vi "User@CallVIWait__Parameter.vi"(1 "ParamterIn":string) -> (0 "ParamterOut":string)   [LabVIEW 2019]
uses:
  MainFrame/Global.vi
panel:
  in  "VI":string(combo)
  in  "Confirm":bool
  # "User@CallVIWait $VI"
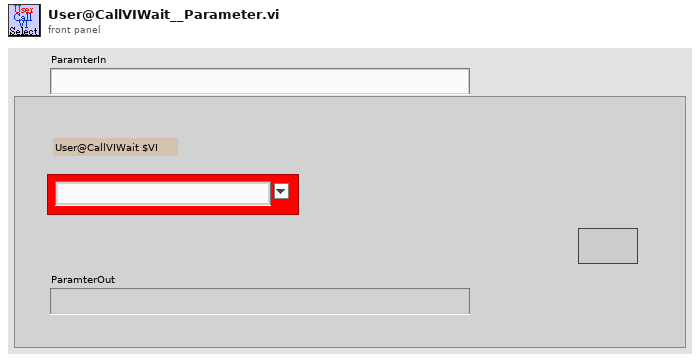
[diagram p1: front panel]
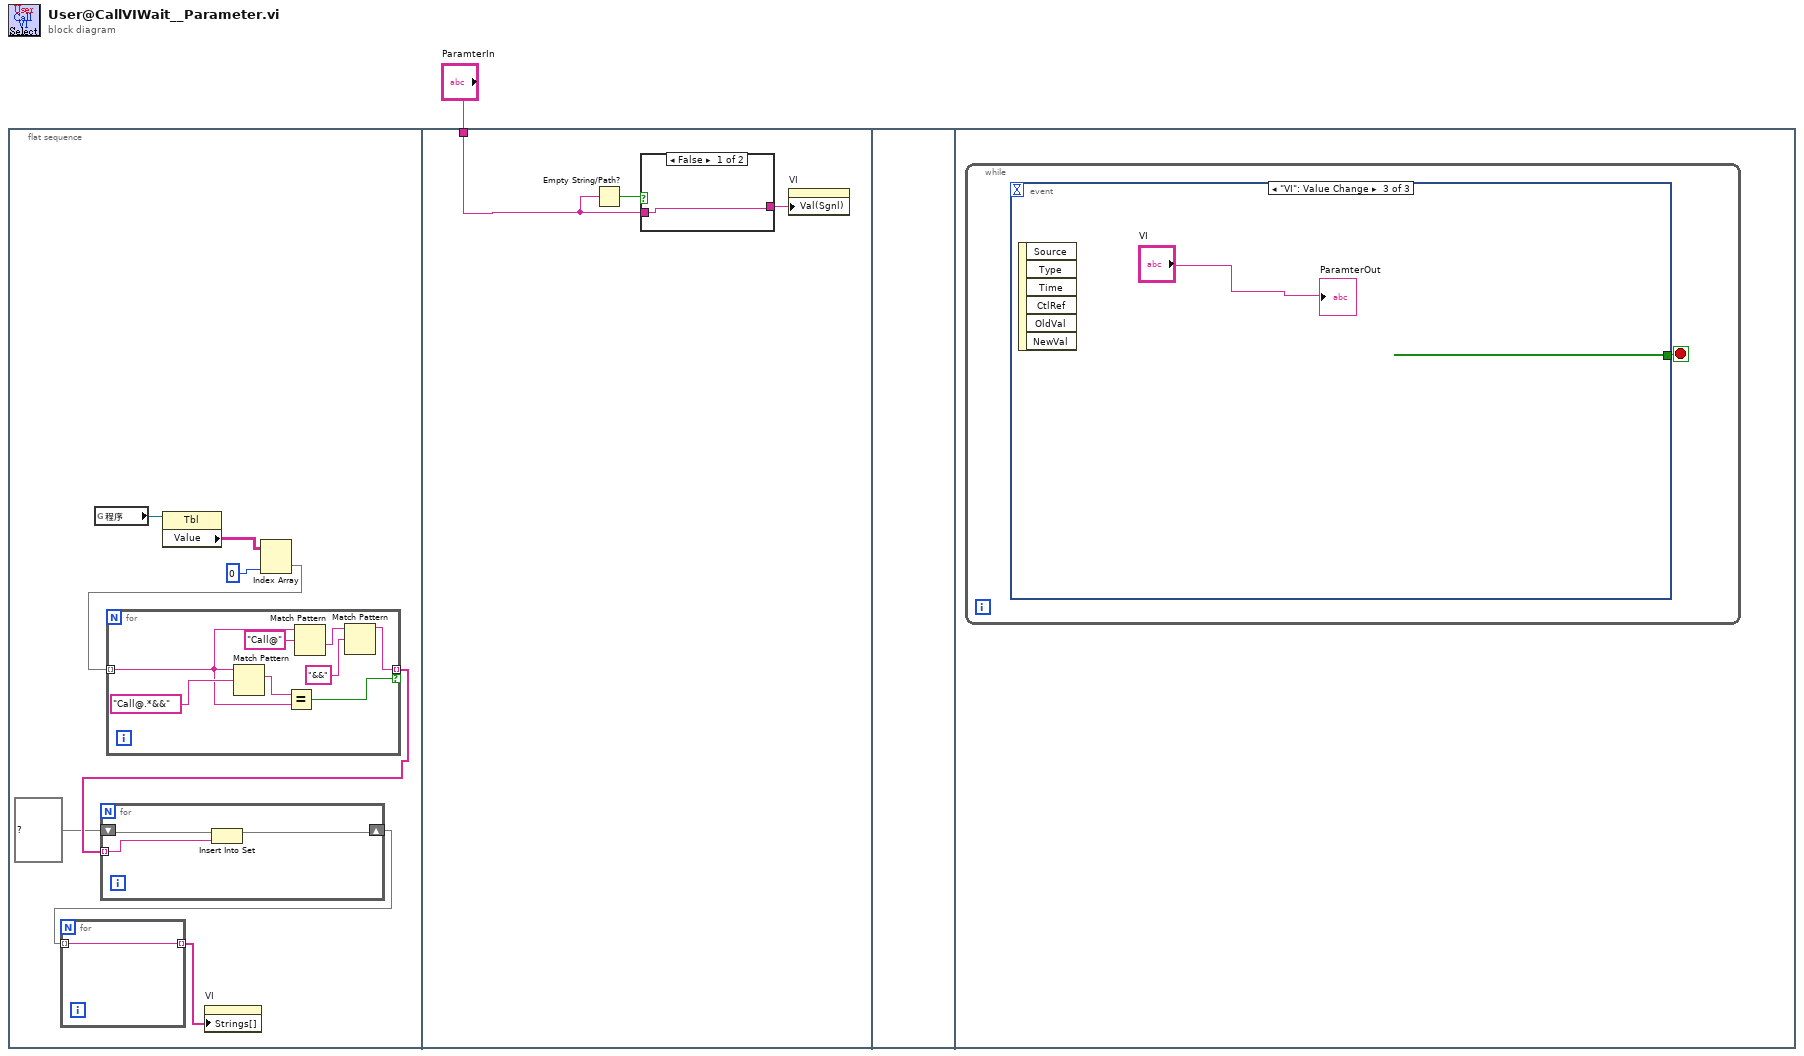
[diagram p0: block diagram]
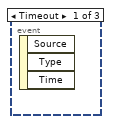
[diagram p3: hidden frame]
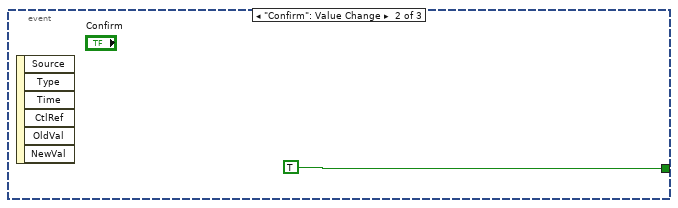
[diagram p4: hidden frame]
diagram:
  n1 = flat-sequence {
    tunnel: "ParamterIn" -> [w22]
    frame #0 {
      n2 = global read "Global.vi" "程序"() -> (w9:refnum<vi>)
      n3 = property class="Tbl"(reference=w9) -> ("Value"=w8:string[][])  [unwired: 1 in, 2 out]
      n4 = Index Array(array=w8, index (col)=0 ("index (row)")) -> (element=w6:string[])  [unwired: 1 in]
      n5 = for {
        tunnel: w6 -> [w18] mode=indexing
        tunnel: [w14] -> w5 mode=indexing if=w19
        n6 = Match Pattern(string=w18, regular expression="Call@.*&&") -> (match substring=w20:string)  [unwired: 1 in, 3 out]
        n7 = Equal?(x=w20, y=w18) -> (x = y?=w19:bool)
        n8 = Match Pattern(string=w18, regular expression="Call@") -> (after substring=w16:string)  [unwired: 1 in, 3 out]
        n9 = Match Pattern(string=w16, regular expression="&&") -> (before substring=w14:string)  [unwired: 1 in, 3 out]
      }
      n10 = for {
        tunnel: w5 -> [w12] mode=indexing
        shift-right: [w11] -> w3
        shift-left: set{string} {} ("set") -> [w13]
        n11 = Insert Into Set(10:w12, 11:w13) -> (3:w11:set{string})  [unwired: 1 out]
      }
      n12 = for {
        tunnel: [w10] -> w2 mode=indexing
        tunnel: w3 -> [w10] mode=indexing
      }
      n13 = property on="VI" class="CmbBox"("Strings[]"=w2) -> ()  [unwired: 2 in, 2 out]
    }
    frame #1 {
      n14 = Empty String/Path?(string/path=w22) -> (empty?=w24:bool)
      n15 = case shown="False" w24 {
        tunnel: w22 -> [w25 w26]
        tunnel: [w25 w26] -> w23
        frame False {
        }
        frame True {
        }
      }
      n16 = property on="VI" class="CmbBox"("Val(Sgnl)"=w23) -> ()  [unwired: 2 in, 2 out]
    }
    frame #2 {
    }
    frame #3 {
      n17 = while {
        stop <- w27 stop-if-true
        n18 = event shown="[2] \"VI\": Value Change" {
          selector: _ -> [_ _ _]
          dyn-events: _ -> [_ _ _]
          timeout: _ -> [_ _ _]
          tunnel: [_ TRUE _] -> w27
          event Timeout {
            n19 = event-data() -> ()  [unwired: 1 in, 3 out]
          }
          event "Confirm": Value Change {
            n20 = event-data() -> ()  [unwired: 1 in, 6 out]
          }
          event "VI": Value Change {
            n21 = event-data() -> ()  [unwired: 1 in, 6 out]
            "ParamterOut" <- "VI"
          }
        }
      }
    }
  }
